vi "Generate Command Frame Vectors.vi"(0 "RFFE RegRead Command in":refnum<class "RFFE RegRead Command.lvclass">, 11 "error in (no error)":errorcluster) -> (4 "RFFE RegRead Command out":refnum<class "RFFE RegRead Command.lvclass">, 6 "Command Frame Vectors":string[](array[string]), 15 "error out":errorcluster)   [LabVIEW 2018, in "MIPI RFFE API.lvlib" / "RFFE RegRead Command.lvclass"]
uses:
  RFFE RegRead Command.lvclass
  Standard Command/RFFE Standard Command.lvclass
  MIPI RFFE API.lvlib
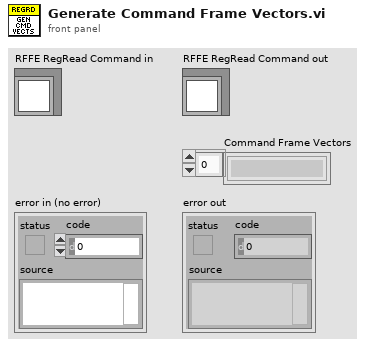
[diagram p1: front panel]
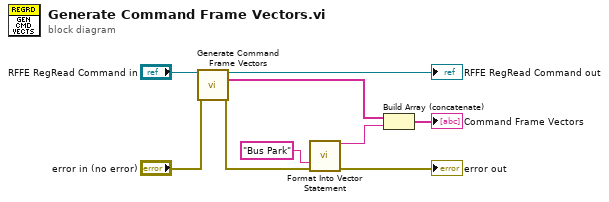
[diagram p0: block diagram]
diagram:
  n1 = call-parent "Generate Command Frame Vectors.vi"("RFFE Standard Command in"="RFFE RegRead Command in", "error in (no error)"="error in (no error)") -> ("RFFE Standard Command out"=→"RFFE RegRead Command out":refnum<class "RFFE RegRead Command.lvclass">, "Command Frame Vectors"=w2:string[], "error out"=w6:errorcluster)  [unwired: 11 in]
  n2 = call "Format Into Vector Statement.vi"("Comment"="Bus Park", "error in (no error)"=w6) -> ("Vector Statement"=w3:string, "error out"=→"error out":errorcluster)  [unwired: 12 in]
  n3 = Build Array (concatenate)(w2, w3) -> (→"Command Frame Vectors":string[])
